vi "detect modules.vi"() -> (0 "error out":errorcluster, 1 "device models":string[](array[string]), 2 "passed?":bool)   [LabVIEW 2014, in "tests.lvlib"]
uses:
  tests.lvlib
  classes/SysCfg Device/SysCfg Device.lvclass
  classes/Controller/Controller.lvclass
  <vilib>/utf/common/utf_test_result.ctl
  <vilib>/utf/NI_UnitTestFramework.lvlib
  <vilib>/utf/common/utf_vi_tag.ctl
  <vilib>/utf/common/utf_test_comparison_operators.ctl
  <vilib>/utf/common/utf_test_result_failure.ctl
  <vilib>/utf/common/utf_test_result_troll.ctl
  classes/Chassis/Chassis.lvclass
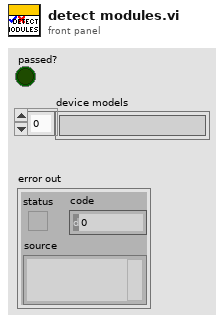
[diagram p1: front panel]
types:
  T1 = typedef "SMI.lvlib/Device.lvclass/login credentials.ctl" = cluster{"device class":string, "hostname":string, "IP address":string, "username":string, "password":string}
  T2 = typedef "SMI.lvlib/Chassis.lvclass/chassis and module information.ctl" = cluster{"chassis":T3, "modules":T4[]}
  T3 = typedef "SMI.lvlib/Chassis.lvclass/chassis information.ctl" = cluster{"resource name":string, "vendor name":string, "product name":string, "product ID":u16, "serial number":string, "number of slots":i32, "device class":string}
  T4 = typedef "SMI.lvlib/Module.lvclass/module information.ctl" = cluster{"vendor name":string, "product name":string, "product ID":u16, "serial number":string}
  T5 = typedef "NI_UnitTestFramework.lvlib/utf_test_result_troll.ctl" = cluster{"time elapsed [ms]":u32, "result (test)":T6, "result (parameters)":T7[]}
  T6 = typedef "NI_UnitTestFramework.lvlib/utf_test_result.ctl" = enum16{"Passed", "Failed", "Error", "Skipped", "Not Processed"}
  T7 = typedef "NI_UnitTestFramework.lvlib/utf_test_result_failure.ctl" = cluster{"result":T6, "error message":string, "parameter name":string, "parameter value":variant, "parameters":variant[], "comparison":T8, "requirement ID":string, "VI":T9, "Used Vector Name":string}
  T8 = typedef "NI_UnitTestFramework.lvlib/utf_test_comparison_operators.ctl" = enum16{"=", "!=", ">", ">=", "<", "<=", "range", "symmetric tolerance", "asymmetric tolerance", "string contains", "string not contain", "array size", "string length", "array range", "by element", "array range (limit array)", "user-defined", "array contains", "array not contain", "vector length", "= (elm)", "!= (elm)", "= (case insensitive)", "!= (case insensitive)"}
  T9 = typedef "NI_UnitTestFramework.lvlib/utf_vi_tag.ctl" = enum16{"Setup VI", "VI under Test", "Teardown VI"}
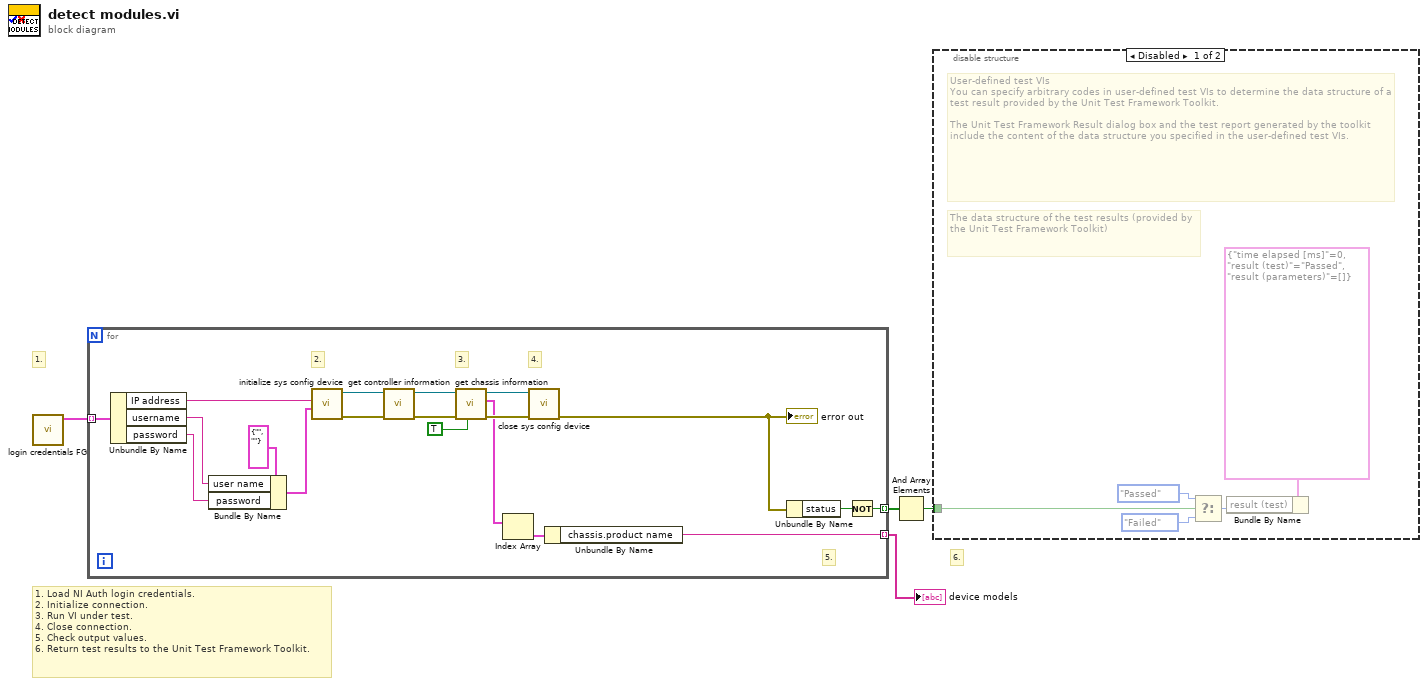
[diagram p0: block diagram]
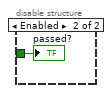
[diagram p2: hidden frame]
diagram:
  # "1."
  # "6."
  # "1. Load NI Auth login credentials.\n2. Initialize connection.\n3. Run VI under test.\n4. Close connection.\n5. Check output values.\n6. Return test results to the Unit Test Framework Toolkit."
  n1 = call "login credentials FG.vi"() -> ("login credentials"=w2:T1[])  [unwired: 10 in, 1 out]
  n2 = for {
    tunnel: [w21] -> w3 mode=indexing
    tunnel: w2 -> [w12] mode=indexing
    tunnel: [w5] -> w1 mode=indexing
    # "4."
    # "2."
    # "3."
    # "5."
    n3 = Unbundle By Name(w12) -> ("IP address"=w11:string, "username"=w9:string, "password"=w10:string)
    n4 = Bundle By Name(cluster=cluster{"user name":string, "password":string} {"user name"="", "password"=""} ("login"), "user name"=w9, "password"=w10) -> (w13:cluster{"user name":string, "password":string})
    n5 = call "initialize sys config device.vi"("login"=w13, "IP address (localhost)"=w11) -> ("error out"=w23:errorcluster, "controller out"=w22:refnum<class "Controller.lvclass">)  [unwired: 8 in]
    n6 = call "get controller information.vi"("error in"=w23, "controller in"=w22) -> ("error out"=w20:errorcluster, "controller out"=w18:refnum<class "Controller.lvclass">)  [unwired: 7 in, 1 out]
    n7 = call "get chassis information.vi"("detect modules (T)"=TRUE, "error in"=w20, "controller in"=w18) -> ("error out"=w19:errorcluster, "local chassis"=w7:T2[], "controller out"=w17:refnum<class "Controller.lvclass">)  [unwired: 5 in, 1 out]
    n8 = Index Array(array=w7) -> (element=w6:T2)  [unwired: 1 in]
    n9 = call "close sys config device.vi"("error in"=w19, "controller in"=w17) -> ("error out"=w8:errorcluster)  [unwired: 8 in, 1 out]
    "error out" <- w8
    n10 = Unbundle By Name(w6) -> ("chassis.product name"=w5:string)
    n11 = Unbundle By Name(w8) -> ("status"=w16:bool)
    n12 = Not(x=w16) -> (.not. x?=w21:bool)
  }
  "device models" <- w1
  n13 = And Array Elements(Boolean array=w3) -> (logical AND=w4:bool)
  n14 = disable-structure shown="Disabled" {
    disable-tunnel: w4 -> [w24 w29]
    frame Disabled {
      # "User-defined test VIs\nYou can specify arbitrary codes in user-defined test VIs to determine the data structure of a test result provided by the Unit Test Framework Toolkit.\n\nThe Unit Test Framework Result dialog box and the test report generated by the toolkit include the content of the data structure you specified in the user-defined test VIs."
      # "The data structure of the test results (provided by the Unit Test Framework Toolkit)"
      n15 = Select(t=utf_test_result."Passed" ("Result (Test)"), s=w24, f=utf_test_result."Failed" ("Result (Test)")) -> (s? t:f=w28:T6)
      n16 = Bundle By Name(cluster=T5 {"time elapsed [ms]"=0, "result (test)"=enum."Passed", "result (parameters)"=[]} ("Constant"), "result (test)"=w28) -> ()  [unwired: 1 out]
    }
    frame Enabled {
      "passed?" <- w29
    }
  }
